vi "Acquire.vi"(6 "Acquisition":refnum<queue>, 7 "Longueur d'onde":dbl, 8 "error in (no error)":errorcluster, 9 "Data Queue":refnum<queue>, 10 "Data Notifier":refnum<notifier>, 11 "Data Stream":dbl[](array[numeric])) -> (0 "error out":errorcluster, 3 "Disconnected":bool=TRUE)   [LabVIEW 2022 SP3, in "Acquisition.lvlib"]
doc: "Perform the acquisition. Replace the contents of this diagram with calls to acquisition hardware."
uses:
  Acquisition.lvlib
  support/Message Queue/Message Cluster.ctl
  support/Message Queue/Message Queue.lvlib
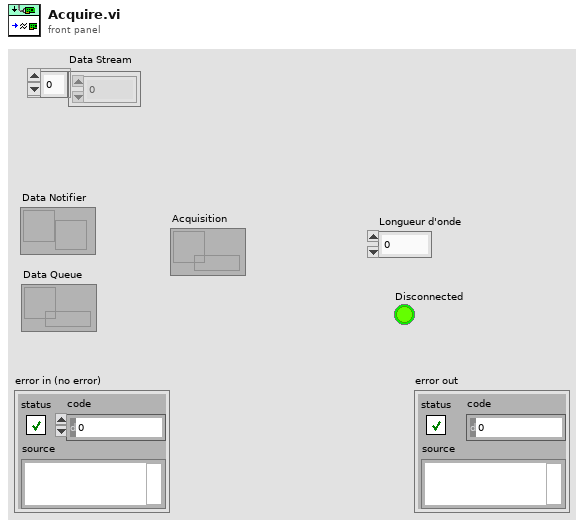
[diagram p1: front panel]
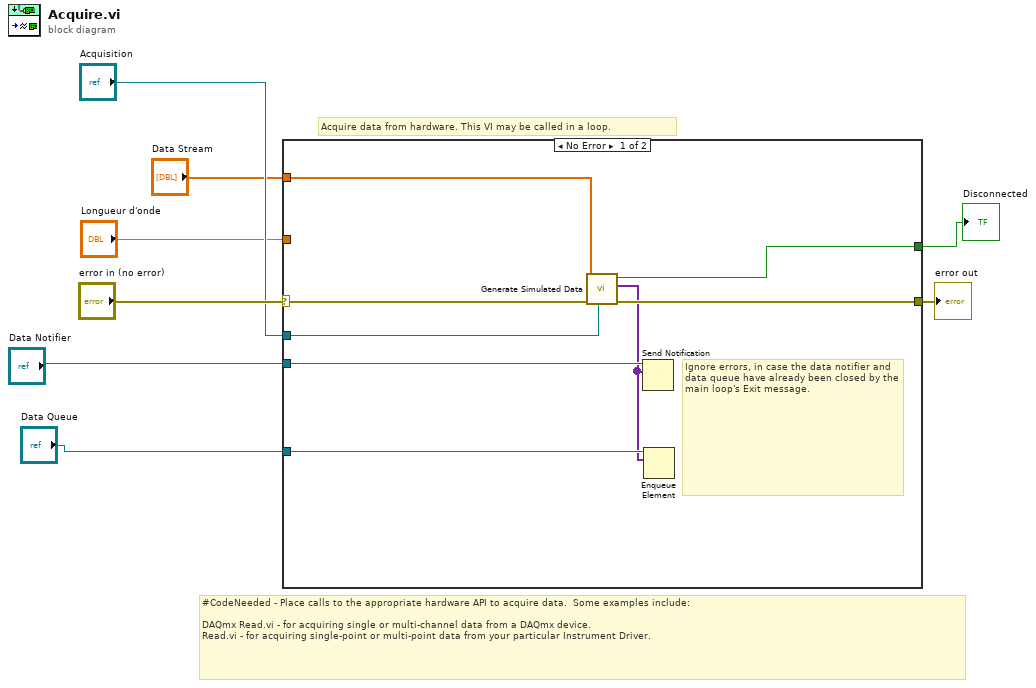
[diagram p0: block diagram]
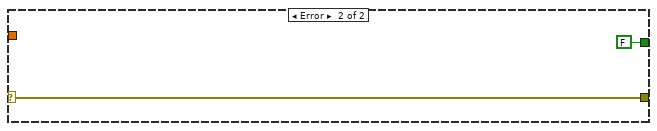
[diagram p2: hidden frame]
diagram:
  # "Acquire data from hardware. This VI may be called in a loop."
  # "#CodeNeeded - Place calls to the appropriate hardware API to acquire data.  Some examples include:\n\nDAQmx Read.vi - for acquiring single or multi-channel data from a DAQmx device.\nRead.vi - for acquiring single-point or multi-point data from your particular Instrument Driver."
  n1 = case shown="No Error" "error in (no error)" {
    selector: "error in (no error)" -> [w16 w18]
    tunnel: [w13 w18] -> w7
    tunnel: "Data Notifier" -> [w15 _]
    tunnel: "Data Queue" -> [w14 _]
    tunnel: "Acquisition" -> [w12 _]
    tunnel: "Longueur d'onde" -> [_ _]
    tunnel: [w10 FALSE ("Disconnected")] -> w2
    tunnel: "Data Stream" -> [w9 _]
    frame No Error {
      # "Ignore errors, in case the data notifier and data queue have already been closed by the main loop's Exit message."
      n2 = call "Generate Simulated Data.vi"("Acquisition"=w12, "error in (no error)"=w16, "Data Stream"=w9) -> ("error out"=w13:errorcluster, "Data Out"=w11:variant[], "Disconnected"=w10:bool)  [unwired: 6 in]
      n3 = Send Notification(notification=w11, notifier=w15) -> ()  [unwired: 1 in, 2 out]
      n4 = Enqueue Element(queue=w14, element=w11) -> ()  [unwired: 2 in, 3 out]
    }
    frame Error {
    }
  }
  "error out" <- w7
  "Disconnected" <- w2
